vi "仁科电流状态解析.vi"(11 "传感器状态输入":u16[](array[numeric])) -> (3 "传感器状态输出":T1)   [LabVIEW 2016, in "环境动力监测库.lvlib" / "空调库.lvlib"]
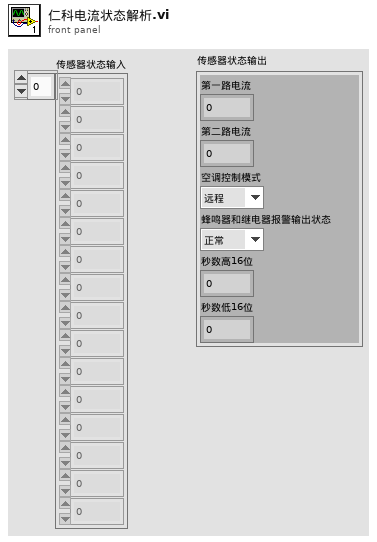
[diagram p1: front panel]
types:
  T1 = cluster{"第一路电流":u16, "第二路电流":u16, "空调控制模式":enum16{"远程", "自动"}, "蜂鸣器和继电器报警输出状态":enum16{"正常", "报警"}, "秒数高16位":u16, "秒数低16位":u16}
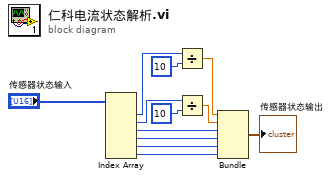
[diagram p0: block diagram]
diagram:
  n1 = Index Array(array="传感器状态输入") -> (element #1=w11:u16, element #2=w9:u16, element #3=w5:u16, element #4=w4:u16, element #5=w3:u16, element #6=w2:u16)  [unwired: 6 in]
  n2 = Divide(x=w11, y=u16 10) -> (x/y=w7:dbl)
  n3 = Divide(x=w9, y=u16 10) -> (x/y=w6:dbl)
  n4 = Bundle(w7, w6, w5, w4, w3, w2) -> (→"传感器状态输出":cluster{dbl, dbl, u16, u16, u16, u16})  [unwired: 1 in]
